vi "IIR Filter.vi"() -> ()   [LabVIEW 2020]
uses:
  <vilib>/Analysis/3filter.llb/Filter Passband Type.ctl
  <vilib>/Analysis/3filter.llb/Butterworth Filter (DBL).vi
  <vilib>/Analysis/3filter.llb/Chebyshev Filter (DBL).vi
  <vilib>/Analysis/3filter.llb/Inverse Chebyshev Filter (DBL).vi
  <vilib>/Analysis/3filter.llb/Bessel Filter (DBL).vi
  <vilib>/Analysis/3filter.llb/Elliptic Filter (DBL).vi
  <vilib>/Analysis/3filter.llb/IIR Filter (DBL).vi
  <vilib>/measure/NI_MABase.lvlib
  <vilib>/Analysis/NI_AALBase.lvlib
panel:
  in  "g":dbl(knob) scale=0.0..10.0
  in  "N":u32(slide) scale=0.0..10.0
  in  "Filtru Prototip":dbl(knob)=1.0 min=0.0 max=4.0 step=1.0 scale=0.0..4.0
  in  "Frecv. de taiere sup\nPt. trece-sus si tr-banda":dbl(slide)=0.45000000000000007 step=1.0 scale=0.0..1000.0
  out "Filtru IIR":dbl[](graph)
  out "Filtru prototip":dbl[](graph)
  in  "Ordinul":i32=2
  in  "Frecv. de taiere inf\nPt. trece-jos si op-banda":dbl(slide)=0.12500000000000006 step=1.0 scale=0.0..1000.0
  in  "Frecventa de esantionare":dbl=1.0 format="%0.2f"
  in  "Tipul filtrului portotip":T1
  out "Semnal cu Zgomot":waveform(dbl)(graph)
  in  "stop":bool
  in  "Zgomot":dbl(slide) step=1.0 scale=0.0..10.0
  out "Semnal initial":waveform(dbl)(graph)
  in  "Sampling Info":cluster{"Frecventa":dbl, "Nr. esantioane":dbl}={"Frecventa"=1000.0, "Nr. esantioane"=1000.0} {"Frecventa" format="%.2p"}
  in  "Amplitudinea":dbl(slide) step=1.0 scale=0.0..10.0
  in  "Frecventa":dbl(slide) step=100.0 scale=0.0..1000.0
  in  "Tipul semnalului":T2(ring)
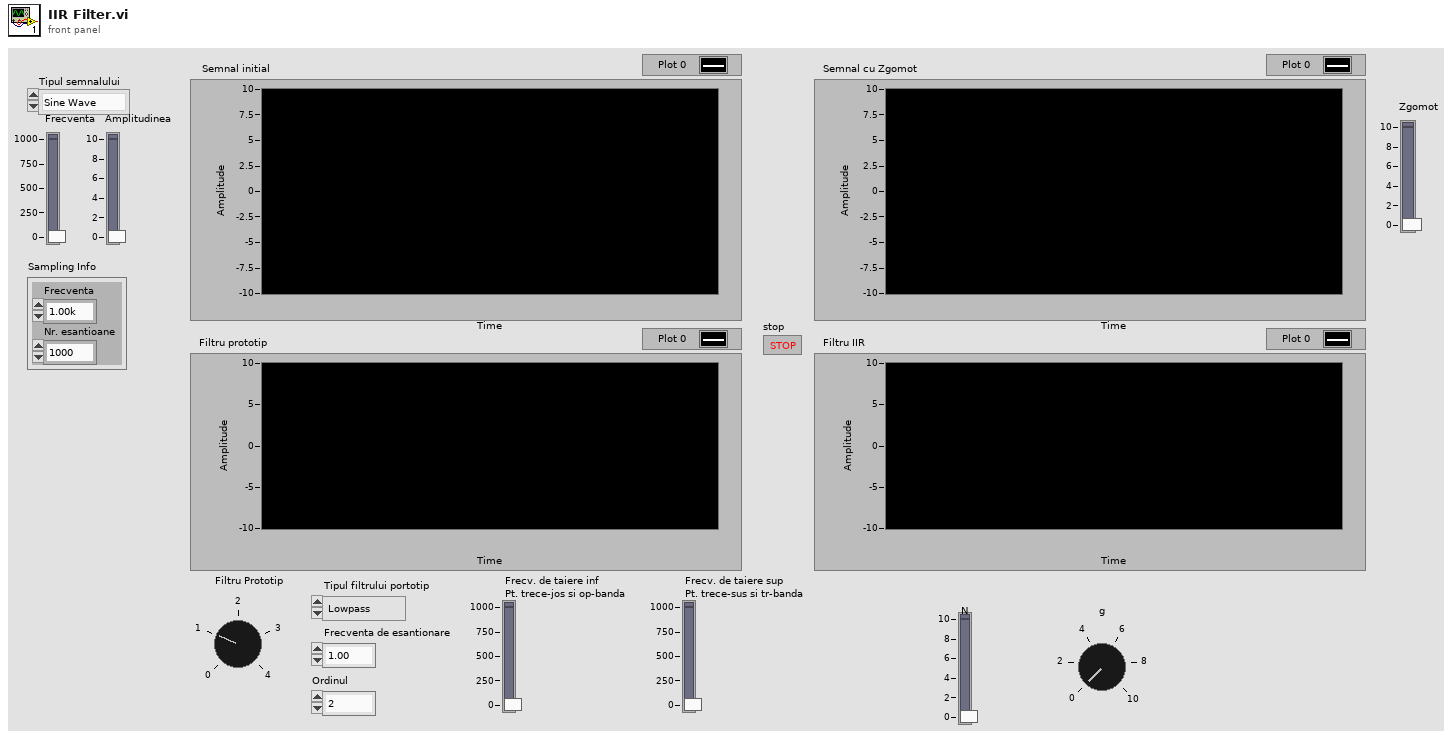
[diagram p1: front panel]
types:
  T1 = typedef "NI_AALBase.lvlib/Filter Passband Type.ctl" = enum32{"Lowpass", "Highpass", "Bandpass", "Bandstop"}
  T2 = enum16{"Sine Wave", "Triangle Wave", "Square Wave", "Sawtooth Wave"}
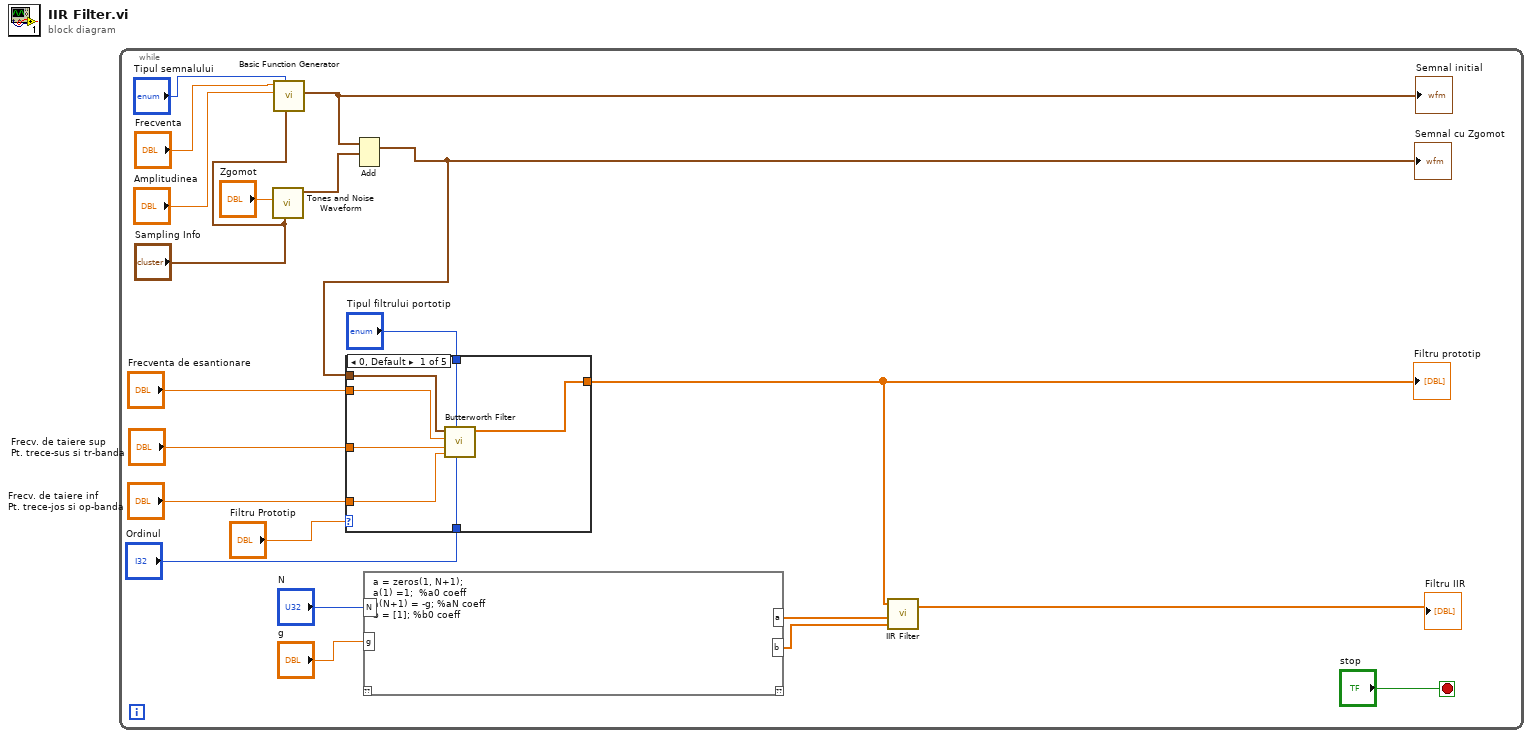
[diagram p0: block diagram]
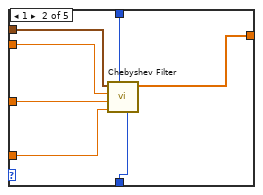
[diagram p2: hidden frame]
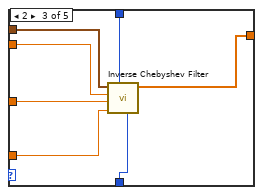
[diagram p3: hidden frame]
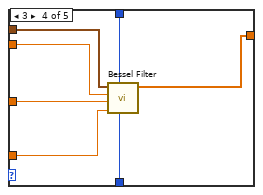
[diagram p4: hidden frame]
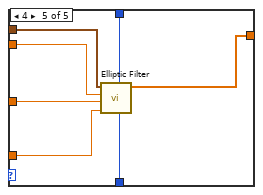
[diagram p5: hidden frame]
diagram:
  n1 = while {
    stop <- "stop" stop-if-true
    n2 = call <vilib>:"Tones and Noise Waveform.vi"("sampling info"="Sampling Info", "noise (rms)"="Zgomot") -> ("signal out"=w15:waveform(dbl))  [unwired: 8 in, 1 out]
    n3 = call <vilib>:"Basic Function Generator.vi"("sampling info"="Sampling Info", "signal type"="Tipul semnalului", "amplitude"="Amplitudinea", "frequency"="Frecventa") -> ("signal out"=w16:waveform(dbl))  [unwired: 5 in, 2 out]
    "Semnal initial" <- w16
    n4 = Add(1:w15, 2:w16) -> (0:w2:waveform(dbl))  [unwired: 1 in, 1 out]
    "Semnal cu Zgomot" <- w2
    n5 = case shown="0, Default" "Filtru Prototip" {
      tunnel: "Tipul filtrului portotip" -> [w28 w35 w42 w49 w56]
      tunnel: "Ordinul" -> [w23 w30 w41 w48 w55]
      tunnel: "Frecventa de esantionare" -> [w26 w33 w39 w45 w52]
      tunnel: "Frecv. de taiere sup\nPt. trece-sus si tr-banda" -> [w25 w32 w38 w44 w51]
      tunnel: "Frecv. de taiere inf\nPt. trece-jos si op-banda" -> [w24 w31 w37 w43 w50]
      tunnel: w2 -> [w27 w34 w40 w46 w53]
      tunnel: [w22 w29 w36 w47 w54] -> w1
      frame 0, Default {
        n6 = call-poly <vilib>:"Butterworth Filter.vi"("order"=w23, "filter type"=w28, "low cutoff freq: fl"=w24, "high cutoff freq: fh"=w25, "sampling freq: fs"=w26, "X"=w27) -> ("Filtered X"=w22:dbl[])  [unwired: 2 in, 1 out]
      }
      frame 1 {
        n7 = call-poly <vilib>:"Chebyshev Filter.vi"("order"=w30, "filter type"=w35, "low cutoff freq: fl"=w31, "high cutoff freq: fh"=w32, "sampling freq: fs"=w33, "X"=w34) -> ("Filtered X"=w29:dbl[])  [unwired: 4 in, 1 out]
      }
      frame 2 {
        n8 = call-poly <vilib>:"Inverse Chebyshev Filter.vi"("order"=w41, "filter type"=w42, "low cutoff freq: fl"=w37, "high cutoff freq: fh"=w38, "sampling freq: fs"=w39, "X"=w40) -> ("Filtered X"=w36:dbl[])  [unwired: 4 in, 1 out]
      }
      frame 3 {
        n9 = call-poly <vilib>:"Bessel Filter.vi"("order"=w48, "filter type"=w49, "low cutoff freq: fl"=w43, "high cutoff freq: fh"=w44, "sampling freq: fs"=w45, "X"=w46) -> ("Filtered X"=w47:dbl[])  [unwired: 2 in, 1 out]
      }
      frame 4 {
        n10 = call-poly <vilib>:"Elliptic Filter.vi"("order"=w55, "filter type"=w56, "low cutoff freq: fl"=w50, "high cutoff freq: fh"=w51, "sampling freq: fs"=w52, "X"=w53) -> ("Filtered X"=w54:dbl[])  [unwired: 4 in, 1 out]
      }
    }
    "Filtru prototip" <- w1
    n11 = script code="a = zeros(1, N+1);\na(1) =1;  %a0 coeff\na(N+1) = -g; %aN coeff\nb = [1]; %b0 coeff"("N"="N", "g"="g") -> ("a"=w6:dbl[], "b"=w5:dbl[])  [unwired: 1 in, 1 out]
    n12 = call-poly <vilib>:"IIR Filter.vi"("Forward Coefficients"=w5, "Reverse Coefficients"=w6, "X"=w1) -> ("Filtered X"=→"Filtru IIR":dbl[])  [unwired: 1 in, 1 out]
  }
